vi "LM3Sxxxx_GPIO_Config.vi"(8 "error in (no error)":errorcluster, 10 "Config Data":string[](array[string]), 11 "interrupt name":string) -> (0 "error out":errorcluster, 3 "Interrupt Configuration":string[](array[string]))   [LabVIEW 2011]
doc: "Select the interrupt configuration for each pin on the GPIO port. Each pin can be configured independently, but all pins on a GPIO port will share the same interrupt handler.\n\nThe <b>Interrupt Type</b> determines the condition under which the pin will generate an interrupt. You can choose to interrupt on either or both edges, or on a high or low level. Leave this setting at None for any pins that are not used for generating interrupts.\n\nThe <b>Input Type</b> determines if the pin is a normal input or if pull-up or pull-down circuits are enabled. The correct setting is dependent on the design of the board. Leave this at Normal if you are not sure of the correct setting."
panel:
  in  "help":bool
  in  "Input7":u32(ring) items=["Normal"=0, "Weak Pull-up"=32768, "Weak Pull-down"=128]
  in  "Input6":u32(ring) items=["Normal"=0, "Weak Pull-up"=16384, "Weak Pull-down"=64]
  in  "Input5":u32(ring) items=["Normal"=0, "Weak Pull-up"=8192, "Weak Pull-down"=32]
  in  "Input4":u32(ring) items=["Normal"=0, "Weak Pull-up"=4096, "Weak Pull-down"=16]
  in  "Input3":u32(ring) items=["Normal"=0, "Weak Pull-up"=2048, "Weak Pull-down"=8]
  in  "Input2":u32(ring) items=["Normal"=0, "Weak Pull-up"=1024, "Weak Pull-down"=4]
  in  "Input1":u32(ring) items=["Normal"=0, "Weak Pull-up"=512, "Weak Pull-down"=2]
  in  "Input0":u32(ring) items=["Normal"=0, "Weak Pull-up"=256, "Weak Pull-down"=1]
  out "Port":string
  in  "Pin 0":u32(ring) items=["None"=0, "Rising Edge"=16777472, "Falling Edge"=16777216, "Both Edges"=16777217, "Low Level"=16842752, "High Level"=16843008]
  in  "Pin 1":u32(ring) items=["None"=0, "Rising Edge"=33554944, "Falling Edge"=33554432, "Both Edges"=33554434, "Low Level"=33685504, "High Level"=33686016]
  in  "Pin 2":u32(ring) items=["None"=0, "Rising Edge"=67109888, "Falling Edge"=67108864, "Both Edges"=67108868, "Low Level"=67371008, "High Level"=67372032]
  in  "Pin 3":u32(ring) items=["None"=0, "Rising Edge"=134219776, "Falling Edge"=134217728, "Both Edges"=134217736, "Low Level"=134742016, "High Level"=134744064]
  in  "Pin 4":u32(ring) items=["None"=0, "Rising Edge"=268439552, "Falling Edge"=268435456, "Both Edges"=268435472, "Low Level"=269484032, "High Level"=269488128]
  in  "Pin 5":u32(ring) items=["None"=0, "Rising Edge"=536879104, "Falling Edge"=536870912, "Both Edges"=536870944, "Low Level"=538968064, "High Level"=538976256]
  in  "Pin 6":u32(ring) items=["None"=0, "Rising Edge"=1073758208, "Falling Edge"=1073741824, "Both Edges"=1073741888, "Low Level"=1077936128, "High Level"=1077952512]
  in  "Pin 7":u32(ring) items=["None"=0, "Rising Edge"=2147516416, "Falling Edge"=2147483648, "Both Edges"=2147483776, "Low Level"=2155872256, "High Level"=2155905024]
  in  "cancel":bool
  in  "ok":bool
  # "Interrupt\nType"
  # "Input\nType"
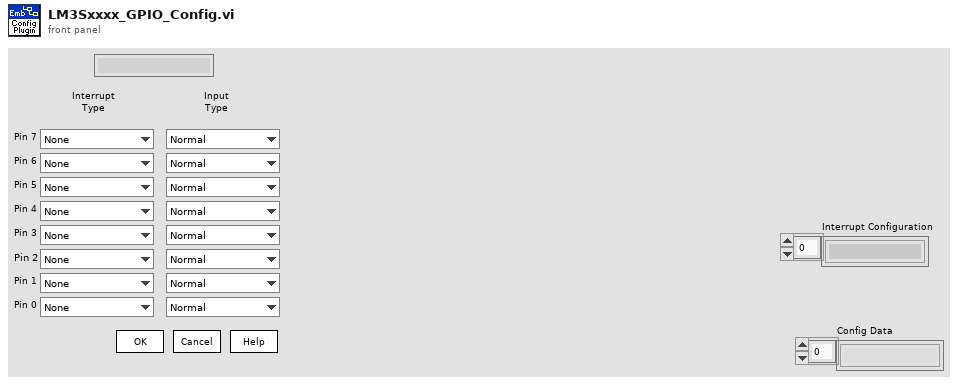
[diagram p1: front panel]
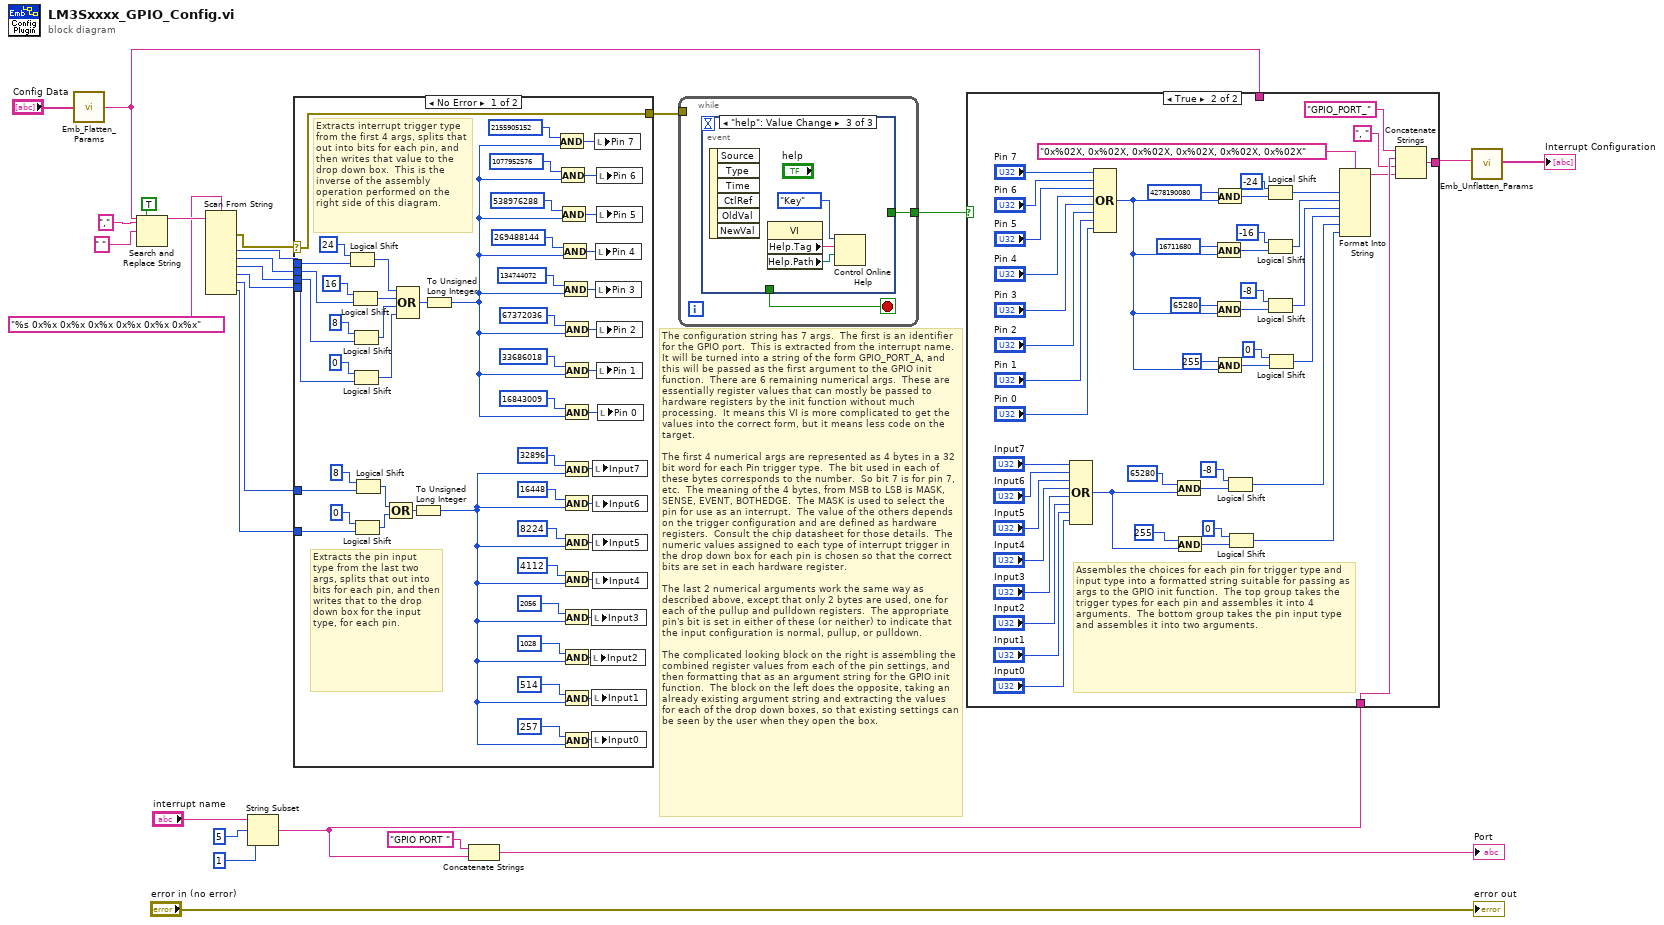
[diagram p0: block diagram]
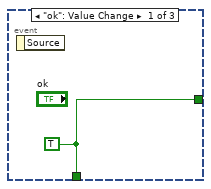
[diagram p4: hidden frame]
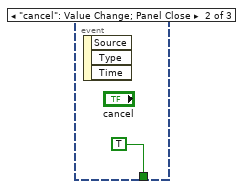
[diagram p5: hidden frame]
diagram:
  # "The configuration string has 7 args.  The first is an identifier for the GPIO port.  This is extracted from the interrupt name.  It will be turned into a string of the form GPIO_PORT_A, and this will be passed as the first argument to the GPIO init function.  There are 6 remaining numerical args.  These are essentially register values that can mostly be passed to hardware registers by the init function without much processing.  It means this VI is more complicated to get the values into the correct form, but it means less code on the target.\n\nThe first 4 numerical args are represented as 4 bytes in a 32 bit word for each Pin trigger type.  The bit used in each of these bytes corresponds to the number.  So bit 7 is for pin 7, etc.  The meaning of the 4 bytes, from MSB to LSB is MASK, SENSE, EVENT, BOTHEDGE.  The MASK is used to select the pin for use as an interrupt.  The value of the others depends on the trigger configuration and are defined as hardware registers.  Consult the chip datasheet for those details.  The numeric values assigned to each type of interrupt trigger in the drop down box for each pin is chosen so that the correct bits are set in each hardware register.\n\nThe last 2 numerical arguments work the same way as described above, except that only 2 bytes are used, one for each of the pullup and pulldown registers.  The appropriate pin's bit is set in either of these (or neither) to indicate that the input configuration is normal, pullup, or pulldown.\n\nThe complicated looking block on the right is assembling the combined register values from each of the pin settings, and then formatting that as an argument string for the GPIO init function.  The block on the left does the opposite, taking an already existing argument string and extracting the values for each of the drop down boxes, so that existing settings can be seen by the user when they open the box."
  n1 = call "Emb_Flatten_Params.vi"("InitDefaultParams"="Config Data") -> ("String"=w11:string)
  n2 = Search and Replace String(replace all?=TRUE ("replace all? (F)"), input string=w11, search string=",", replace string=" " ("replace string (\"\")")) -> (result string=w15:string)  [unwired: 1 in, 6 out]
  n3 = Scan From String(format string="%s 0x%x 0x%x 0x%x 0x%x 0x%x 0x%x", input string=w15) -> (error out=w8:errorcluster, output 2=w7:i32, output 3=w6:i32, output 4=w5:i32, output 5=w4:i32, output 6=w3:i32, output 7=w2:i32)  [unwired: 2 in, 10 out]
  n4 = String Subset(string="interrupt name", offset (0)=5, length (rest)=1 ("length (rest)")) -> (substring=w19:string)
  n5 = case shown="No Error" w8 {
    selector: w8 -> [w28 w81]
    tunnel: w7 -> [w80 _]
    tunnel: w6 -> [w75 _]
    tunnel: w5 -> [w74 _]
    tunnel: w4 -> [w73 _]
    tunnel: [w28 w81] -> w17
    tunnel: w3 -> [w49 _]
    tunnel: w2 -> [w48 _]
    frame No Error {
      # "Extracts the pin input type from the last two args, splits that out into bits for each pin, and then writes that to the drop down box for the input type, for each pin."
      # "Extracts interrupt trigger type from the first 4 args, splits that out into bits for each pin, and then writes that value to the drop down box.  This is the inverse of the assembly operation performed on the right side of this diagram."
      n6 = Logical Shift(y=u32 24 ("x"), x=w80) -> (x << y=w72:i32)
      n7 = Logical Shift(y=u32 16 ("x"), x=w75) -> (x << y=w71:i32)
      n8 = Logical Shift(y=u32 8 ("x"), x=w74) -> (x << y=w70:i32)
      n9 = Logical Shift(y=u32 0 ("x"), x=w73) -> (x << y=w69:i32)
      n10 = Logical Shift(y=u32 0 ("x"), x=w48) -> (x << y=w46:i32)
      n11 = Logical Shift(y=u32 8 ("x"), x=w49) -> (x << y=w47:i32)
      n12 = Compound Arithmetic op=OR(w47, w46) -> (w45:i32)
      n13 = Compound Arithmetic op=OR(w72, w71, w70, w69) -> (w68:i32)
      n14 = To Unsigned Long Integer(number=w45) -> (unsigned 32bit integer=w26:u32)
      n15 = To Unsigned Long Integer(number=w68) -> (unsigned 32bit integer=w27:u32)
      n16 = And(x=u32 2155905152, y=w27) -> (x .and. y?=w59:u32)
      n17 = And(x=u32 1077952576, y=w27) -> (x .and. y?=w58:u32)
      n18 = And(x=u32 538976288, y=w27) -> (x .and. y?=w57:u32)
      n19 = And(x=u32 269488144, y=w27) -> (x .and. y?=w56:u32)
      n20 = And(x=u32 134744072, y=w27) -> (x .and. y?=w55:u32)
      n21 = And(x=u32 67372036, y=w27) -> (x .and. y?=w54:u32)
      n22 = And(x=u32 33686018, y=w27) -> (x .and. y?=w53:u32)
      n23 = And(x=u32 16843009, y=w27) -> (x .and. y?=w52:u32)
      n24 = And(x=u32 32896, y=w26) -> (x .and. y?=w36:u32)
      n25 = And(x=u32 16448, y=w26) -> (x .and. y?=w34:u32)
      n26 = And(x=u32 8224, y=w26) -> (x .and. y?=w33:u32)
      n27 = And(x=u32 4112, y=w26) -> (x .and. y?=w32:u32)
      n28 = And(x=u32 2056, y=w26) -> (x .and. y?=w31:u32)
      n29 = And(x=u32 1028, y=w26) -> (x .and. y?=w30:u32)
      n30 = And(x=u32 514, y=w26) -> (x .and. y?=w29:u32)
      n31 = And(x=u32 257, y=w26) -> (x .and. y?=w35:u32)
      n32 = local write "Input2"(w30) -> ()
      n33 = local write "Input3"(w31) -> ()
      n34 = local write "Input1"(w29) -> ()
      n35 = local write "Input0"(w35) -> ()
      n36 = local write "Input7"(w36) -> ()
      n37 = local write "Input6"(w34) -> ()
      n38 = local write "Input5"(w33) -> ()
      n39 = local write "Input4"(w32) -> ()
      n40 = local write "Pin 7"(w59) -> ()
      n41 = local write "Pin 4"(w56) -> ()
      n42 = local write "Pin 3"(w55) -> ()
      n43 = local write "Pin 6"(w58) -> ()
      n44 = local write "Pin 5"(w57) -> ()
      n45 = local write "Pin 2"(w54) -> ()
      n46 = local write "Pin 1"(w53) -> ()
      n47 = local write "Pin 0"(w52) -> ()
    }
    frame Error {
    }
  }
  n48 = Concatenate Strings("GPIO PORT " ("string"), w19) -> (→"Port":string)
  n49 = while {
    tunnel: [w82] -> w18
    tunnel: w17 -> [_]
    stop <- w83 stop-if-true
    n50 = event shown="[2] \"help\": Value Change" {
      selector: _ -> [_ _ _]
      dyn-events: _ -> [_ _ _]
      timeout: _ -> [_ _ _]
      tunnel: [w84 TRUE _] -> w83
      tunnel: [w84 _ _] -> w82
      event "ok": Value Change {
        w84 = TRUE
        n51 = event-data() -> ()  [unwired: 2 out]
      }
      event "cancel": Value Change; Panel Close {
        n52 = event-data() -> ()  [unwired: 4 out]
      }
      event "help": Value Change {
        n53 = event-data() -> ()  [unwired: 7 out]
        n54 = property class="VI"() -> ("Help.Tag"=w86:string, "Help.Path"=w87:path)  [unwired: 2 in, 2 out]
        n55 = Control Online Help(2:w87, 3:w86, 4:enum16{"Contents", "Key", "Close"}."Key" ("Operation")) -> ()  [unwired: 1 in, 1 out]
      }
    }
  }
  n56 = case shown="True" w18 {
    tunnel: w19 -> [_ w119]
    tunnel: [w89 w108] -> w10
    tunnel: w11 -> [w89 _]
    frame False {
    }
    frame True {
      # "Assembles the choices for each pin for trigger type and input type into a formatted string suitable for passing as args to the GPIO init function.  The top group takes the trigger types for each pin and assembles it into 4 arguments.  The bottom group takes the pin input type and assembles it into two arguments."
      n57 = Compound Arithmetic op=OR("Input7", "Input6", "Input5", "Input4", "Input3", "Input2", "Input1", "Input0") -> (w107:u32)
      n58 = Compound Arithmetic op=OR("Pin 7", "Pin 6", "Pin 5", "Pin 4", "Pin 3", "Pin 2", "Pin 1", "Pin 0") -> (w126:u32)
      n59 = And(x=u32 65280, y=w107) -> (x .and. y?=w103:u32)
      n60 = And(x=u32 255, y=w107) -> (x .and. y?=w105:u32)
      n61 = And(x=u32 16711680, y=w126) -> (x .and. y?=w114:u32)
      n62 = And(x=u32 65280, y=w126) -> (x .and. y?=w112:u32)
      n63 = And(x=u32 4278190080, y=w126) -> (x .and. y?=w116:u32)
      n64 = And(x=u32 255, y=w126) -> (x .and. y?=w110:u32)
      n65 = Logical Shift(y=-8 ("x"), x=w103) -> (x << y=w91:u32)
      n66 = Logical Shift(y=0 ("x"), x=w105) -> (x << y=w92:u32)
      n67 = Logical Shift(y=-24 ("x"), x=w116) -> (x << y=w124:u32)
      n68 = Logical Shift(y=-16 ("x"), x=w114) -> (x << y=w123:u32)
      n69 = Logical Shift(y=-8 ("x"), x=w112) -> (x << y=w122:u32)
      n70 = Logical Shift(y=0 ("x"), x=w110) -> (x << y=w121:u32)
      n71 = Format Into String(format string="0x%02X, 0x%02X, 0x%02X, 0x%02X, 0x%02X, 0x%02X", w124, w123, w122, w121, w91, w92) -> (resulting string=w117:string)  [unwired: 2 in, 1 out]
      n72 = Concatenate Strings("GPIO_PORT_" ("string"), w119, ", " ("string"), w117) -> (w108:string)
    }
  }
  n73 = call "Emb_Unflatten_Params.vi"("String"=w10) -> ("InitDefaultParams"=→"Interrupt Configuration":string[])  [unwired: 10 out]
  "error out" <- "error in (no error)"
